vi "H5Tget_ebias.vi"(6 "error in (no error)":errorcluster, 9 "HDF5 Ref":T1) -> (0 "error out":errorcluster, 2 "ebias":u32, 3 "HDF5 Ref out":T1)   [LabVIEW 2017]
doc: "Retrieves the exponent bias of a floating-point type."
uses:
  <vilib>/UPVI/lvhdf5/library.llb/HDF5 Ref.ctl
  <vilib>/UPVI/lvhdf5/hdf5.dll
panel:
  # "LVHDF5 Toolkit\nCopyright (c) 2005-2013 by Jason D. Sommerville\nCopyright (c) 2014 by UPVI, LLC.\n\nThis use and distribution of this file is governed by the terms found in \nLICENSE.txt distributed with this toolkit and installed at\n <user.lib>\\_lvhdf5\\LICENSE.txt"
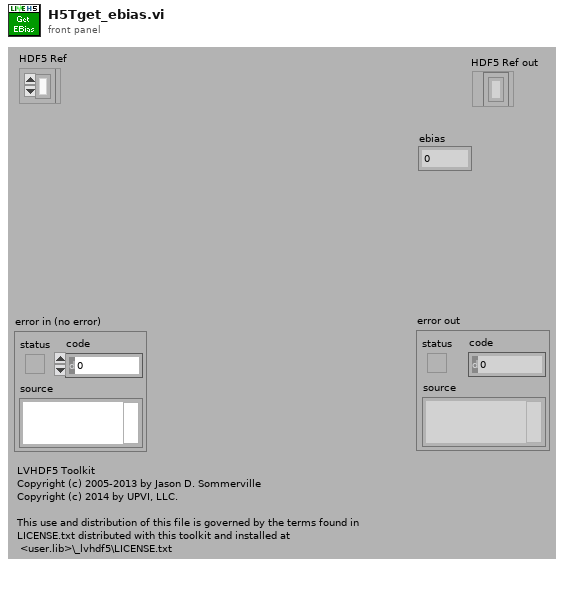
[diagram p1: front panel]
types:
  T1 = typedef "HDF5 Ref.ctl" = refnum<k1>
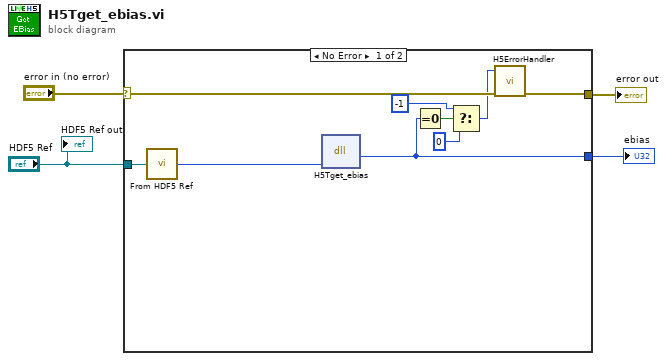
[diagram p0: block diagram]
diagram:
  n1 = case shown="No Error" "error in (no error)" {
    selector: "error in (no error)" -> [w13 w14]
    tunnel: [w12 w14] -> w3
    tunnel: "HDF5 Ref" -> [w11 _]
    tunnel: [w6 _] -> w1
    frame No Error {
      n2 = call <vilib>:"From HDF5 Ref.vi"("HDF5 Ref"=w11) -> ("I32"=w10:i32)
      n3 = dll-call lib="C:/Program Files/National Instruments/LabVIEW 2017/vi.lib/UPVI/lvhdf5/hdf5.dll" fn="H5Tget_ebias"("loc_id"=w10) -> ("return type"=w6:u64)  [unwired: 4 in, 2 out]
      n4 = Equal To 0?(x=w6) -> (x = 0?=w9:bool)
      n5 = Select(t=-1 ("I32"), s=w9, f=0 ("I32")) -> (s? t:f=w7:i32)
      n6 = call <vilib>:"H5ErrorHandler.vi"("error in (no error)"=w13, "herr_t"=w7) -> ("error out"=w12:errorcluster)  [unwired: 3 in, 4 out]
    }
    frame Error {
    }
  }
  "error out" <- w3
  "ebias" <- w1
  "HDF5 Ref out" <- "HDF5 Ref"
